vi "Z Aux Trace Out.vi"(8 "error in (no error)":errorcluster caption="错误输入（无错误）", 10 "para1":cluster{} caption="空簇", 11 "cText":string) -> (0 "error out":errorcluster caption="错误输出")   [LabVIEW 2015, in "zauxdll.lvlib"]
doc: "#define ZAUX_TRACE(cText,a) ZAux_TraceOut(\"%s,L:%u,\"cText\"\\r\\n\",__FILE__,(unsigned int)__LINE__,a)\n#define ZAUX_WARN(cText,a) ZAux_TraceOut(\"%s,L:%u,\"cText\"\\r\\n\",__FILE__,(unsigned int)__LINE__,a)\n#define ZAUX_ERROR(cText,a) ZAux_TraceOut(\"Error:%s,L:%u,\"cText\"\\r\\n\",__FILE__,(unsigned int)__LINE__,a)\n#define ZAUX_ERROR2(cText,a,b) ZAux_TraceOut(\"Error:%s,L:%u,\"cText\"\\r\\n\",__FILE__,(unsigned int)__LINE__,a,b)\n\n#else\n\n#define ZAUX_TRACE(cText,a)\n#define ZAUX_WARN(cText,a)\n#define ZAUX_ERROR(cText,a)\n#define ZAUX_ERROR2(cText,a,b)\n\n#endif\n\nvoid ZAux_TraceOut(const char * cText, ...);"
uses:
  zauxdll.lvlib
  zauxdll.dll
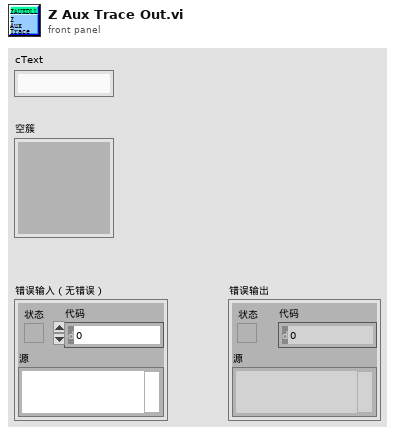
[diagram p1: front panel]
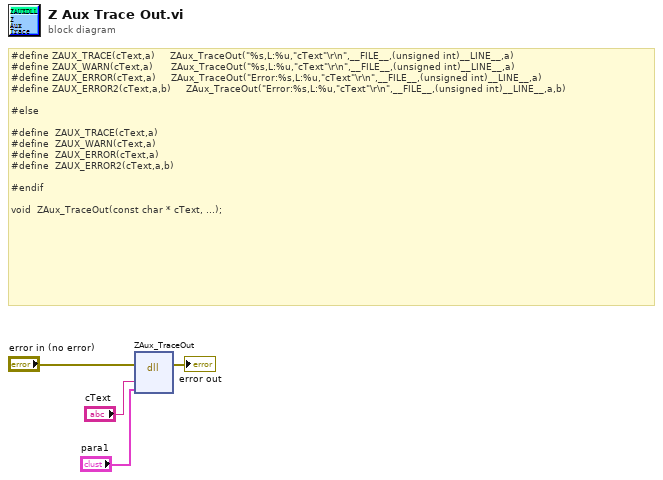
[diagram p0: block diagram]
diagram:
  # "#define ZAUX_TRACE(cText,a)     ZAux_TraceOut(\"%s,L:%u,\"cText\"\\r\\n\",__FILE__,(unsigned int)__LINE__,a)\n#define ZAUX_WARN(cText,a)      ZAux_TraceOut(\"%s,L:%u,\"cText\"\\r\\n\",__FILE__,(unsigned int)__LINE__,a)\n#define ZAUX_ERROR(cText,a)     ZAux_TraceOut(\"Error:%s,L:%u,\"cText\"\\r\\n\",__FILE__,(unsigned int)__LINE__,a)\n#define ZAUX_ERROR2(cText,a,b)     ZAux_TraceOut(\"Error:%s,L:%u,\"cText\"\\r\\n\",__FILE__,(unsigned int)__LINE__,a,b)\n\n#else\n\n#define  ZAUX_TRACE(cText,a)\n#define  ZAUX_WARN(cText,a)\n#define  ZAUX_ERROR(cText,a)\n#define  ZAUX_ERROR2(cText,a,b)\n\n#endif\n\nvoid  ZAux_TraceOut(const char * cText, ...);"
  n1 = dll-call lib="C:/Users/VIC/Desktop/GOGORO_Oringnal - Panasonic/system/LLB/zmotion/zaux/zauxdll.*" fn="ZAux_TraceOut"(error in="error in (no error)", "cText"="cText", "para1"="para1") -> (error out=→"error out":errorcluster)  [unwired: 5 in, 1 out]
